vi "Read stopMessage.vi"(8 "error in (no error)":errorcluster, 11 "MsgUETaskChannel in":refnum<class "MsgQueueTaskChannel.lvclass">) -> (0 "error out":errorcluster, 2 "stopMessage":string="stop", 3 "MsgUETaskChannel out":refnum<class "MsgQueueTaskChannel.lvclass">)   [LabVIEW 2023, in "TLC_Daemon.lvlib" / "MsgQueueTaskChannel.lvclass"]
uses:
  MsgQueueTaskChannel.lvclass
  MsgQueueTaskChannel.lvclass/MsgQueueTaskChannel.ctl
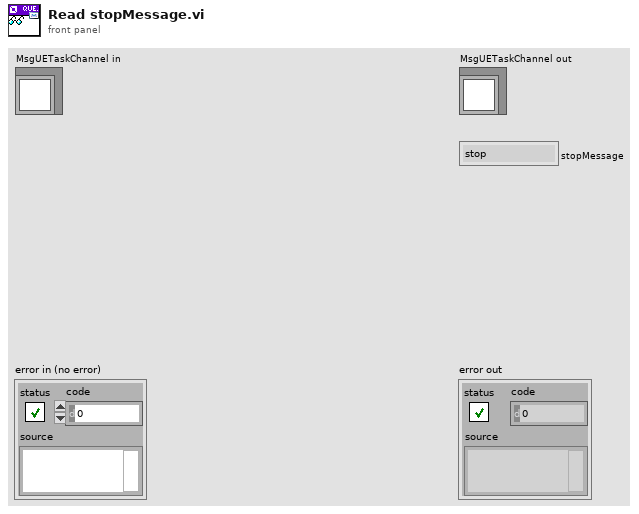
[diagram p1: front panel]
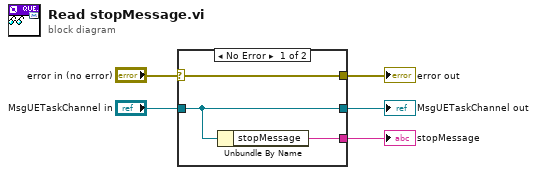
[diagram p0: block diagram]
diagram:
  n1 = case shown="No Error" "error in (no error)" {
    selector: "error in (no error)" -> [w8 w9]
    tunnel: [w8 w9] -> w4
    tunnel: [w7 w10] -> w2
    tunnel: "MsgUETaskChannel in" -> [w7 w10]
    tunnel: [w6 _] -> w1
    frame No Error {
      n2 = Unbundle By Name(w7) -> ("stopMessage"=w6:string)
    }
    frame Error {
    }
  }
  "error out" <- w4
  "MsgUETaskChannel out" <- w2
  "stopMessage" <- w1
